vi "SelectCommand.vi"(11 "Select Command":T1="SEARCHADDRH") -> (3 "Command":u32)   [LabVIEW 2014, in "Driver_interaction.lvlib" / "Dali_usb_tridonics.lvclass"]
doc: "Select command from an Enum and get the decimal command."
uses:
  Dali_usb_tridonics.lvclass
  Controls/Commands enum.ctl
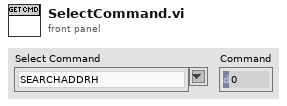
[diagram p1: front panel]
types:
  T1 = typedef "Driver_interaction.lvlib/Dali_usb_tridonics.lvclass/Commands enum.ctl" = string
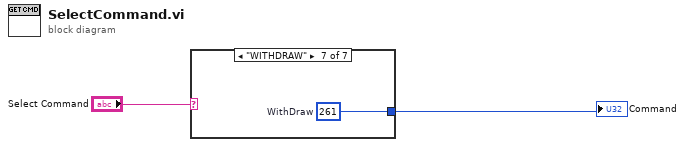
[diagram p0: block diagram]
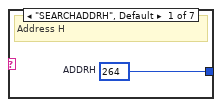
[diagram p2: hidden frame]
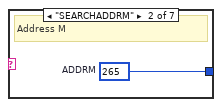
[diagram p3: hidden frame]
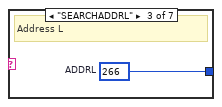
[diagram p4: hidden frame]
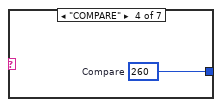
[diagram p5: hidden frame]
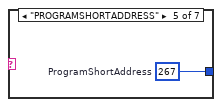
[diagram p6: hidden frame]
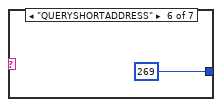
[diagram p7: hidden frame]
diagram:
  n1 = case shown="\"WITHDRAW\"" "Select Command" {
    tunnel: [w3 w4 w5 w6 w7 u32 269 ("ADDRL") w9] -> w1
    frame "SEARCHADDRH", Default {
      w3 = u32 264  # ADDRH
      # "Address H"
    }
    frame "SEARCHADDRM" {
      w4 = u32 265  # ADDRM
      # "Address M"
    }
    frame "SEARCHADDRL" {
      w5 = u32 266  # ADDRL
      # "Address L"
    }
    frame "COMPARE" {
      w6 = u32 260  # Compare
    }
    frame "PROGRAMSHORTADDRESS" {
      w7 = u32 267  # ProgramShortAddress
    }
    frame "QUERYSHORTADDRESS" {
    }
    frame "WITHDRAW" {
      w9 = u32 261  # WithDraw
    }
  }
  "Command" <- w1
